vi "Set Properties.vi"(8 "error in (no error)":errorcluster, 10 "Class Properties":T1 {"Mode" items=["Operator"=0, "Engineering"=1, "Verification"=6]}, 11 "App Properties in":refnum<class "App Properties.lvclass">) -> (0 "error out":errorcluster, 3 "App Properties out":refnum<class "App Properties.lvclass">)   [LabVIEW 2017, in "Application.lvlib" / "App Properties.lvclass"]
uses:
  App Properties.lvclass
  Class/typedefs/Test Info -- Cluster.ctl
  Class/Application.lvclass
  Class Properties -- Cluster.ctl
  Golden Board/Class/Golden Board.lvclass
  Test Recipe/Class/Test Recipe.lvclass
  UUT Reference -- Cluster.ctl
  Class/typedefs/Op Mode -- Enum.ctl
  Station Config/Class/Station Config.lvclass
  Instruments/Instrument/Class/Instrument.lvclass
  Test Result -- Cluster.ctl
  <vilib>/TSS/ACRObat Test Framework/Classes/Variable Engine/Class/Variable Engine.lvclass
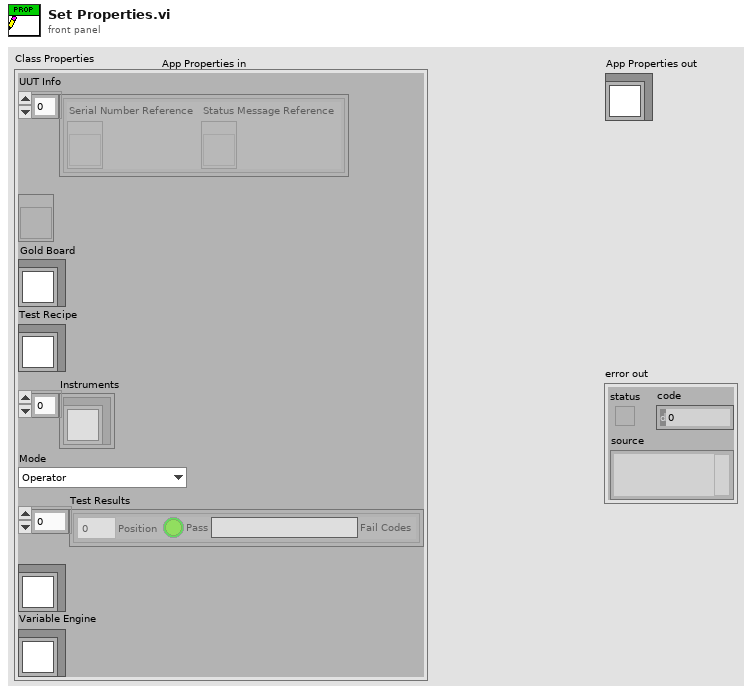
[diagram p1: front panel]
types:
  T1 = typedef "Application.lvlib/App Properties.lvclass/Class Properties -- Cluster.ctl" = cluster{"UUT Info":T2[], "Test Information":refnum<vi>, "Gold Board":refnum<class "Golden Board.lvclass">, "Test Recipe":refnum<class "Test Recipe.lvclass">, "Instruments":refnum<class "Instrument.lvclass">[], "Mode":T3, "Test Results":T4[], "Station Config":refnum<class "Station Config.lvclass">, "Variable Engine":refnum<class "Variable Engine.lvclass">}
  T2 = typedef "Application.lvlib/App Properties.lvclass/UUT Reference -- Cluster.ctl" = cluster{"Serial Number Reference":refnum<vi>, "Status Message Reference":refnum<vi>}
  T3 = typedef "Application.lvlib/Application.lvclass/Op Mode -- Enum.ctl" = u16
  T4 = typedef "Application.lvlib/App Properties.lvclass/Test Result -- Cluster.ctl" = cluster{"Position":i32, "Pass":bool, "Fail Codes":string}
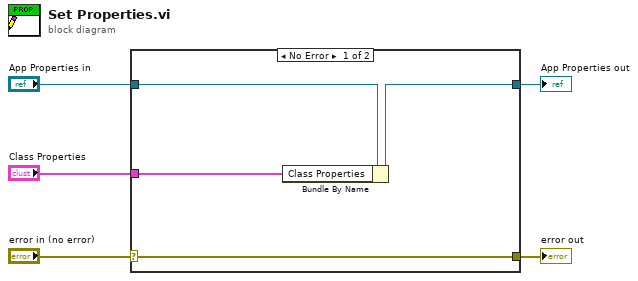
[diagram p0: block diagram]
diagram:
  n1 = case shown="No Error" "error in (no error)" {
    selector: "error in (no error)" -> [w9 w10]
    tunnel: [w9 w10] -> w4
    tunnel: [w7 w11] -> w2
    tunnel: "App Properties in" -> [w8 w11]
    tunnel: "Class Properties" -> [w6 _]
    frame No Error {
      n2 = Bundle By Name(cluster=w8, "Class Properties"=w6) -> (w7:refnum<class "App Properties.lvclass">)
    }
    frame Error {
    }
  }
  "error out" <- w4
  "App Properties out" <- w2
